vi "Update.vi"(8 "error in (no error)":errorcluster, 10 "Message in":refnum<class "UpdateMessage.lvclass">, 11 "Waveform in":refnum<class "Waveform.lvclass">) -> (0 "error out":errorcluster, 3 "Waveform out":refnum<class "Waveform.lvclass">)   [LabVIEW 2012, in "Waveform.lvclass"]
doc: "The update method processes the command 'update'. \n\nThe command 'update' is used for receiving new values to be set to the private data of the class. This could be seen as a public set method for setting new parameters to the private class data."
uses:
  Waveform.lvclass
  <vilib>/Distrio/Murmex/UpdateMessage/UpdateMessage.lvclass
  Waveform.lvclass/Waveform.ctl
  <vilib>/Distrio/Murmex/Murmex/Murmex.lvclass
panel:
  # "This method is called when the UPDATE\ntrigger is sent. \n\nOverride this method when your component needs to\nrespond to this trigger. \n\nCall parent for proper implementation"
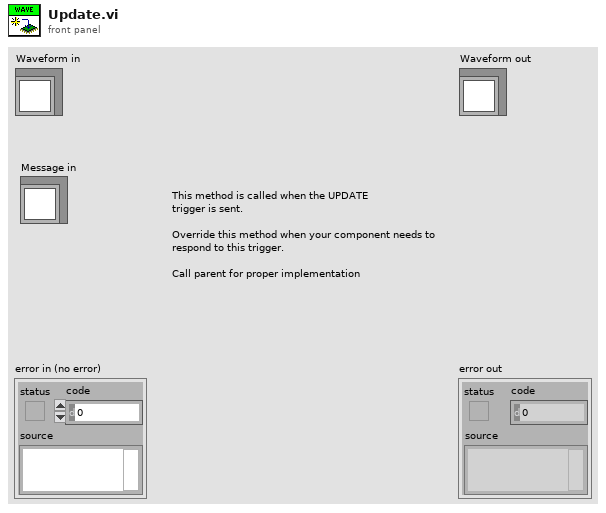
[diagram p1: front panel]
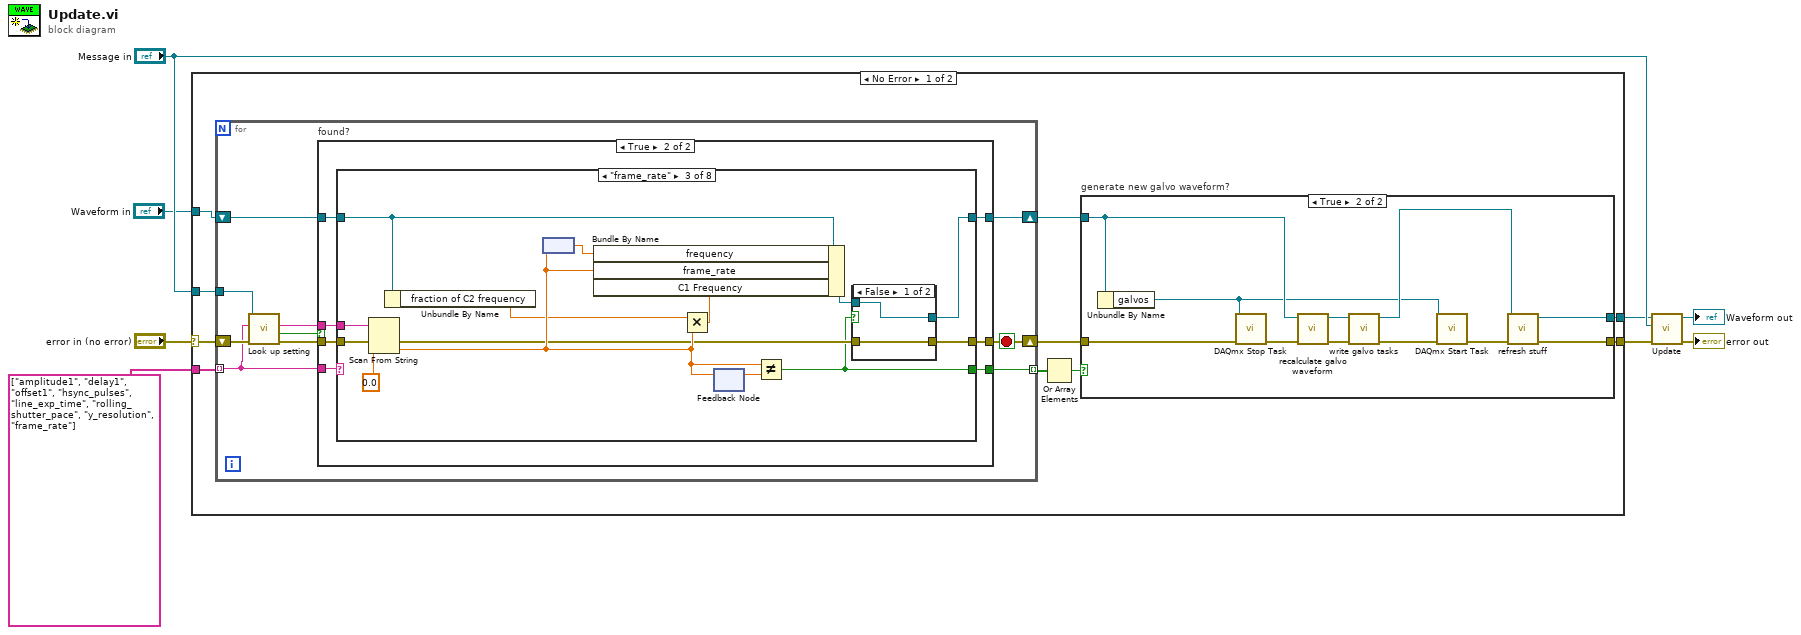
[diagram p0: block diagram]
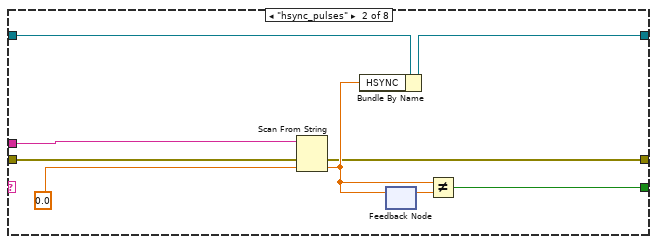
[diagram p5: hidden frame]
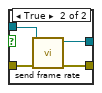
[diagram p6: hidden frame]
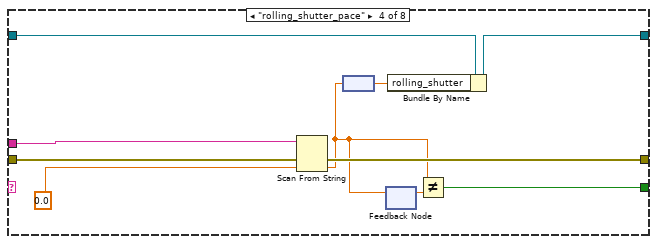
[diagram p7: hidden frame]
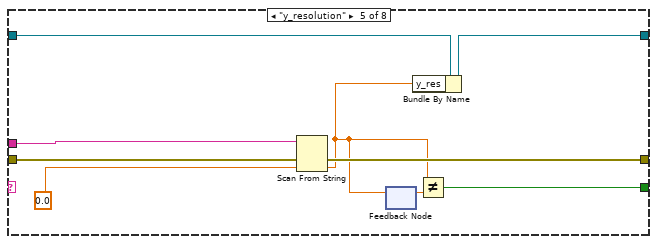
[diagram p8: hidden frame]
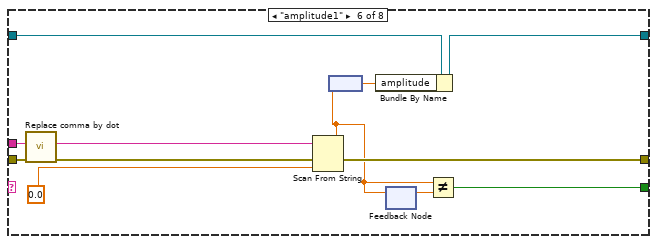
[diagram p9: hidden frame]
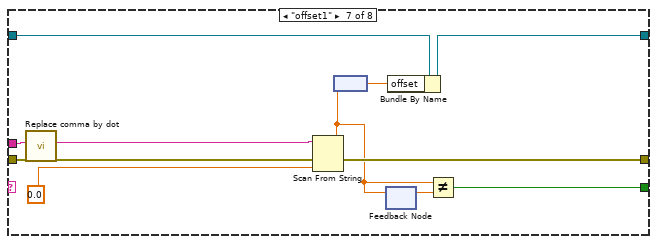
[diagram p10: hidden frame]
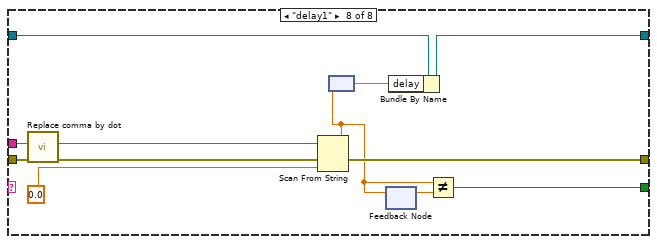
[diagram p11: hidden frame]
diagram:
  n1 = case shown="No Error" "error in (no error)" {
    selector: "error in (no error)" -> [w18 w135]
    tunnel: "Message in" -> [w17 _]
    tunnel: "Waveform in" -> [w16 w136]
    tunnel: string[] ["amplitude1", "delay1", "offset1", "hsync_pulses", "line_exp_time", "rolling_shutter_pace", "y_resolution", "frame_rate"] ("key chains") -> [w15 _]
    tunnel: [w11 w135] -> w3
    tunnel: [w10 w136] -> w2
    frame No Error {
      n2 = for {
        shift-right: [w34] -> w12
        shift-left: w18 -> [w41]
        tunnel: w17 -> [w40]
        shift-right: [w35] -> w9
        shift-left: w16 -> [w39]
        tunnel: w15 -> [w32] mode=indexing
        tunnel: [w33] -> w14 mode=indexing
        stop <- w34 stop-if-true
        n3 = call <vilib>:"Look up setting.vi"("error in (no error)"=w41, "tag name"=w32, "UpdateMessage in"=w40) -> ("error out"=w38:errorcluster, "found?"=w37:bool, "value"=w36:string)  [unwired: 5 in, 1 out]
        n4 = case "found?" shown="True" w37 {
          selector: w37 -> [w42 _]
          tunnel: w39 -> [w44 w50]
          tunnel: w38 -> [w43 w51]
          tunnel: w36 -> [_ w46]
          tunnel: w32 -> [_ w48]
          tunnel: [w44 w49] -> w35
          tunnel: [w43 w47] -> w34
          tunnel: [w42 w45] -> w33
          frame False {
          }
          frame True {
            n5 = case shown="\"frame_rate\"" w48 {
              tunnel: w51 -> [w52 w62 w76 w92 w101 w112 w123 w134]
              tunnel: w50 -> [w53 w61 w69 w91 w100 w111 w122 w133]
              tunnel: [w53 w55 w64 w90 w99 w110 w121 w132] -> w49
              tunnel: [w52 w54 w66 w89 w98 w109 w120 w131] -> w47
              tunnel: w46 -> [_ w60 w75 w88 w97 w103 w114 w125]
              tunnel: [_ w57 w63 w86 w95 w107 w118 w129] -> w45
              frame Default {
              }
              frame "hsync_pulses" {
                n6 = Scan From String(input string=w60, error in=w62, default 1=0.0) -> (error out=w54:errorcluster, output 1=w58:dbl)  [unwired: 2 in, 2 out]
                n7 = Bundle By Name(cluster=w61, "HSYNC"=w58) -> (w55:refnum<class "Waveform.lvclass">)
                n8 = feedback #1() -> (w59:dbl)  [unwired: 1 in]
                n9 = feedback-in #1(w58) -> ()
                n10 = Not Equal?(x=w58, y=w59) -> (x != y?=w57:bool)
              }
              frame "frame_rate" {
                n11 = Scan From String(input string=w75, error in=w76, default 1=0.0) -> (error out=w67:errorcluster, output 1=w71:dbl)  [unwired: 2 in, 2 out]
                n12 = Unbundle By Name(w69) -> ("fraction of C2 frequency"=w68:dbl)
                n13 = node(w71) -> (w70:dbl[unit])
                n14 = Multiply(x=w68, y=w71) -> (x*y=w72:dbl)
                n15 = Bundle By Name(cluster=w69, "frequency"=w70, "frame_rate"=w71, "C1 Frequency"=w72) -> (w65:refnum<class "Waveform.lvclass">)
                n16 = feedback #2() -> (w74:dbl)  [unwired: 1 in]
                n17 = feedback-in #2(w71) -> ()
                n18 = Not Equal?(x=w71, y=w74) -> (x != y?=w63:bool)
                n19 = case shown="False" w63 {
                  tunnel: w67 -> [w77 w82]
                  tunnel: [w77 w81] -> w66
                  tunnel: w65 -> [w78 w80]
                  tunnel: [w78 w79] -> w64
                  frame False {
                  }
                  frame True {
                    n20 = call-dynamic "send frame rate.vi"("error in (no error)"=w82, "Waveform in"=w80) -> ("error out"=w81:errorcluster, "Waveform out"=w79:refnum<class "Waveform.lvclass">)  [unwired: 8 in]
                  }
                }
              }
              frame "rolling_shutter_pace" {
                n21 = Scan From String(input string=w88, error in=w92, default 1=0.0) -> (error out=w89:errorcluster, output 1=w83:dbl)  [unwired: 2 in, 2 out]
                n22 = node(w83) -> (w84:dbl[unit])
                n23 = feedback #3() -> (w87:dbl)  [unwired: 1 in]
                n24 = feedback-in #3(w83) -> ()
                n25 = Bundle By Name(cluster=w91, "rolling_shutter"=w84) -> (w90:refnum<class "Waveform.lvclass">)
                n26 = Not Equal?(x=w83, y=w87) -> (x != y?=w86:bool)
              }
              frame "y_resolution" {
                n27 = Scan From String(input string=w97, error in=w101, default 1=0.0) -> (error out=w98:errorcluster, output 1=w93:dbl)  [unwired: 2 in, 2 out]
                n28 = feedback #4() -> (w96:dbl)  [unwired: 1 in]
                n29 = feedback-in #4(w93) -> ()
                n30 = Bundle By Name(cluster=w100, "y_res"=w93) -> (w99:refnum<class "Waveform.lvclass">)
                n31 = Not Equal?(x=w93, y=w96) -> (x != y?=w95:bool)
              }
              frame "amplitude1" {
                n32 = call <vilib>:"Replace comma by dot.vi"("input string"=w103) -> ("result string"=w102:string)  [unwired: 10 in]
                n33 = Scan From String(input string=w102, error in=w112, default 1=0.0) -> (error out=w109:errorcluster, output 1=w105:dbl)  [unwired: 2 in, 2 out]
                n34 = node(w105) -> (w106:dbl[unit])
                n35 = Bundle By Name(cluster=w111, "amplitude"=w106) -> (w110:refnum<class "Waveform.lvclass">)
                n36 = feedback #5() -> (w108:dbl)  [unwired: 1 in]
                n37 = feedback-in #5(w105) -> ()
                n38 = Not Equal?(x=w105, y=w108) -> (x != y?=w107:bool)
              }
              frame "offset1" {
                n39 = call <vilib>:"Replace comma by dot.vi"("input string"=w114) -> ("result string"=w113:string)  [unwired: 10 in]
                n40 = Scan From String(input string=w113, error in=w123, default 1=0.0) -> (error out=w120:errorcluster, output 1=w116:dbl)  [unwired: 2 in, 2 out]
                n41 = node(w116) -> (w117:dbl[unit])
                n42 = feedback #6() -> (w119:dbl)  [unwired: 1 in]
                n43 = feedback-in #6(w116) -> ()
                n44 = Bundle By Name(cluster=w122, "offset"=w117) -> (w121:refnum<class "Waveform.lvclass">)
                n45 = Not Equal?(x=w116, y=w119) -> (x != y?=w118:bool)
              }
              frame "delay1" {
                n46 = call <vilib>:"Replace comma by dot.vi"("input string"=w125) -> ("result string"=w124:string)  [unwired: 10 in]
                n47 = Scan From String(input string=w124, error in=w134, default 1=0.0) -> (error out=w131:errorcluster, output 1=w127:dbl)  [unwired: 2 in, 2 out]
                n48 = node(w127) -> (w128:dbl[unit])
                n49 = feedback #7() -> (w130:dbl)  [unwired: 1 in]
                n50 = feedback-in #7(w127) -> ()
                n51 = Bundle By Name(cluster=w133, "delay"=w128) -> (w132:refnum<class "Waveform.lvclass">)
                n52 = Not Equal?(x=w127, y=w130) -> (x != y?=w129:bool)
              }
            }
          }
        }
      }
      n53 = Or Array Elements(Boolean array=w14) -> (logical OR=w13:bool)
      n54 = case "generate new galvo waveform?" shown="True" w13 {
        tunnel: w12 -> [w19 w27]
        tunnel: [w19 w28] -> w11
        tunnel: [w20 w29] -> w10
        tunnel: w9 -> [w20 w25]
        frame False {
        }
        frame True {
          n55 = Unbundle By Name(w25) -> ("galvos"=w21:refnum<k21>)
          n56 = call <vilib>:"DAQmx Stop Task.vi"("task/channels in"=w21, "error in"=w27) -> ("error out"=w26:errorcluster)  [unwired: 12 in, 1 out]
          n57 = call-dynamic "recalculate galvo waveform.vi"("error in (no error)"=w26, "Waveform in"=w25) -> ("error out"=w31:errorcluster, "Waveform out"=w30:refnum<class "Waveform.lvclass">)  [unwired: 8 in]
          n58 = call-dynamic "write galvo tasks.vi"("error in (no error)"=w31, "Waveform in"=w30) -> ("error out"=w23:errorcluster, "Waveform out"=w22:refnum<class "Waveform.lvclass">)  [unwired: 8 in]
          n59 = call <vilib>:"DAQmx Start Task.vi"("task/channels in"=w21, "error in"=w23) -> ("error out"=w24:errorcluster)  [unwired: 12 in, 1 out]
          n60 = call-dynamic "refresh stuff.vi"("error in (no error)"=w24, "Waveform in"=w22) -> ("error out"=w28:errorcluster, "Waveform out"=w29:refnum<class "Waveform.lvclass">)  [unwired: 8 in]
        }
      }
    }
    frame Error {
    }
  }
  n61 = call-parent "Update.vi"("error in (no error)"=w3, "Message in"="Message in", "Murmex in"=w2) -> ("error out"=→"error out":errorcluster, "Murmex out"=→"Waveform out":refnum<class "Waveform.lvclass">)  [unwired: 7 in]
